vi "Log.vi"(4 "LogMessage":string, 6 "Type":string, 8 "Error In":errorcluster) -> (0 "Error Out":errorcluster)   [LabVIEW 2017, in "Client.lvlib" / "ClientLogger.lvlib"]
doc: "This VI obtains the MHL-Queue by name, and sends the attached Data including Timestamp to the MHL. This will forward it to the Logging Loop."
uses:
  ClientLogger.lvlib
  Message Queue.lvlib
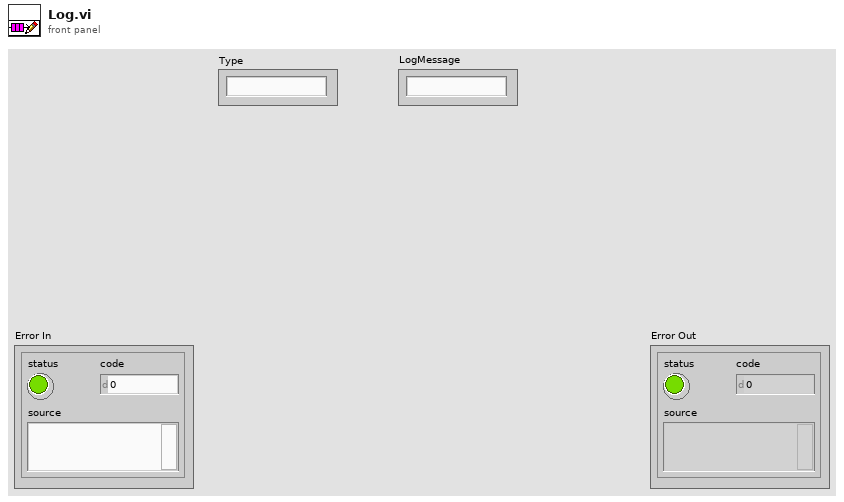
[diagram p1: front panel]
types:
  T1 = cluster{"Message":string, "Message Data":variant}
  T2 = cluster{"Time":timestamp, "Type":string, "LogText":string}
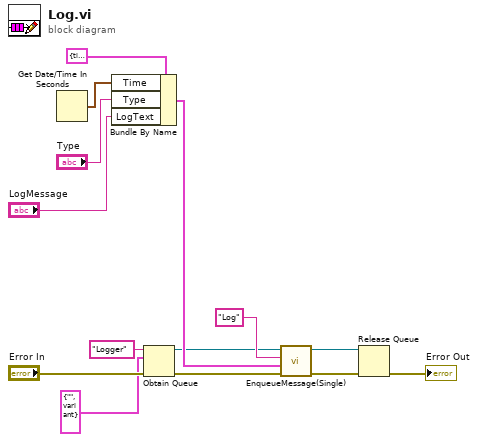
[diagram p0: block diagram]
diagram:
  n1 = Get Date/Time In Seconds() -> (seconds since 1Jan1904=w13:timestamp)
  n2 = Bundle By Name(cluster=T2 {"Time"=timestamp(0 s since 1904-01-01), "Type"="", "LogText"=""} ("LogData"), "Time"=w13, "Type"="Type", "LogText"="LogMessage") -> (w8:T2)
  n3 = Obtain Queue(name (unnamed)="Logger", element data type=T1 {"Message"="", "Message Data"=variant} ("Message Cluster"), error in (no error)="Error In") -> (queue out=w3:refnum<queue>, error out=w6:errorcluster)  [unwired: 2 in, 1 out]
  n4 = call "EnqueueMessage(Single).vi"("error in (no error)"=w6, "Message Data"=w8, "Message"="Log", "Message Queue"=w3) -> ("error out"=w9:errorcluster, "dup Message Queue"=w1:refnum<queue>)  [unwired: 6 in]
  n5 = Release Queue(queue=w1, error in (no error)=w9) -> (error out=→"Error Out":errorcluster)  [unwired: 1 in, 2 out]
